vi "Legendre Polynomial_Pmm (1D).vi"(7 "m":i32, 10 "X In":dbl[](array[numeric])) -> (0 "2m+1":dbl, 2 "X Out":dbl[](array[numeric]), 3 "Pmm(X)":dbl[](array[numeric]))   [LabVIEW 2017, in "NI_AAL_Polynomial.lvlib"]
uses:
  <vilib>/Analysis/NI_AAL_Polynomial.lvlib
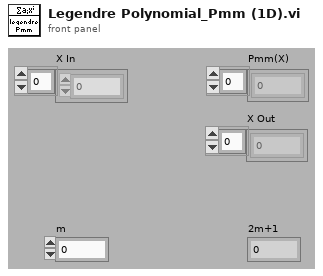
[diagram p1: front panel]
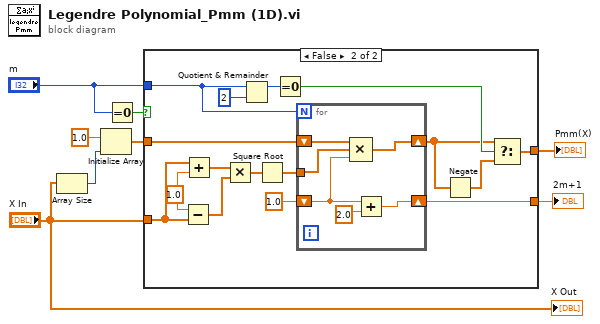
[diagram p0: block diagram]
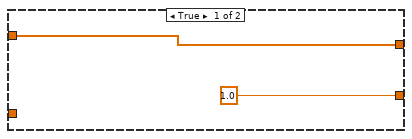
[diagram p2: hidden frame]
diagram:
  n1 = Array Size(array="X In") -> (size(s)=w2:i32)
  n2 = Initialize Array(1.0 ("element"), w2) -> (w4:dbl[])
  n3 = Equal To 0?(x="m") -> (x = 0?=w8:bool)
  n4 = case shown="False" w8 {
    tunnel: "X In" -> [_ w26]
    tunnel: "m" -> [_ w15]
    tunnel: [w9 w14] -> w1
    tunnel: [1.0 ("element") w13] -> w6
    tunnel: w4 -> [w9 w12]
    frame True {
    }
    frame False {
      w25 = 1.0
      n5 = Subtract(x=w25, y=w26) -> (x-y=w23:dbl[])
      n6 = Add(x=w26, y=w25) -> (x+y=w24:dbl[])
      n7 = Multiply(x=w24, y=w23) -> (x*y=w22:dbl[])
      n8 = Quotient & Remainder(x=w15, y=2) -> (x-y*floor(x/y)=w19:i32)  [unwired: 1 out]
      n9 = Square Root(x=w22) -> (sqrt(x)=w11:dbl[])
      n10 = Equal To 0?(x=w19) -> (x = 0?=w18:bool)
      n11 = for {
        N: w15 -> [_]
        shift-right: [w30] -> w13
        shift-left: 1.0 ("element") -> [w27]
        shift-right: [w29] -> w17
        shift-left: w12 -> [w32]
        tunnel: w11 -> [w28]
        n12 = Compound Arithmetic op=MULTIPLY(w32, w28, w27) -> (w29:dbl[])
        n13 = Add(x=w27, y=2.0) -> (x+y=w30:dbl)
      }
      n14 = Negate(x=w17) -> (-x=w16:dbl[])
      n15 = Select(t=w17, s=w18, f=w16) -> (s? t:f=w14:dbl[])
    }
  }
  "2m+1" <- w6
  "Pmm(X)" <- w1
  "X Out" <- "X In"
